vi "PID with MFC Challenge.vi"(8 "error in":errorcluster, 11 "classes in":T1) -> (0 "error out":errorcluster, 3 "classes out":T1)   [LabVIEW 2011]
uses:
  Controls/Class Objects.ctl
  Modules/File/Configuration/Configuration.lvclass
  Modules/Hardware/Power Supply/Power Supply.lvclass
  Modules/Hardware/Mass Flow Controller/Mass Flow Controller.lvclass
  Modules/Hardware/PID/PID.lvclass
  Modules/Hardware/Valve Controller/Valve Controller.lvclass
  Modules/Hardware/Multimeter/Multimeter.lvclass
  Modules/Hardware/Vapour Generator/Vapour Generator.lvclass
  Modules/File/TDMS/TDMS.lvclass
  Controls/User Interface Action.ctl
  Functional Global Data/Device Params Global.ctl
  Functional Global Data/Run Data.ctl
  Controls/TDMS File Handling.ctl
  <vilib>/Platform/TimedLoop/XDataNode/timing_clust.ctl
  <vilib>/Platform/TimedLoop/XDataNode/nitl_modes.ctl
  <vilib>/Platform/TimedLoop/XDataNode/wakeup.ctl
  Modules/File/TDMS/File Level.ctl
  <vilib>/Platform/TimedLoop/XDataNode/XDataNode.xnode
  <vilib>/Platform/TimedLoop/XDataNode/XDNodeRunTimeDep.lvlib
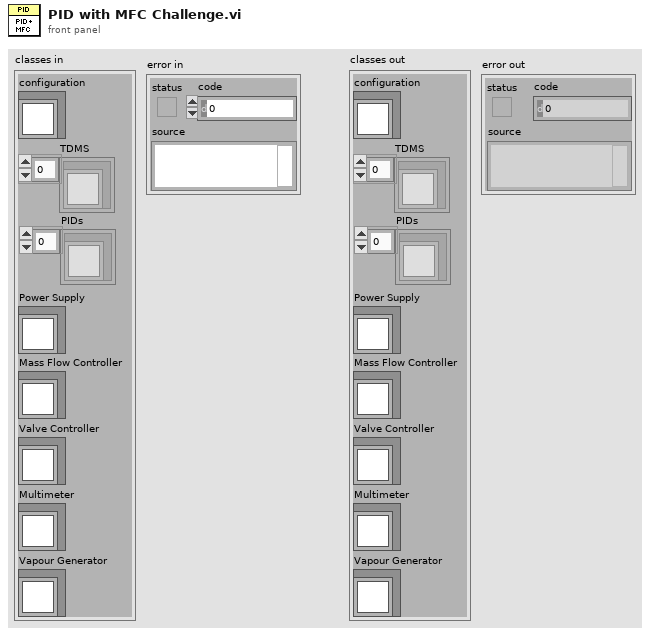
[diagram p1: front panel]
types:
  T1 = typedef "Class Objects.ctl" = cluster{"configuration":refnum<class "Configuration.lvclass">, "TDMS":refnum<class "TDMS.lvclass">[], "Power Supply":refnum<class "Power Supply.lvclass">, "Mass Flow Controller":refnum<class "Mass Flow Controller.lvclass">, "Valve Controller":refnum<class "Valve Controller.lvclass">, "Multimeter":refnum<class "Multimeter.lvclass">, "Vapour Generator":refnum<class "Vapour Generator.lvclass">, "PIDs":refnum<class "PID.lvclass">[]}
  T2 = typedef "User Interface Action.ctl" = enum16{"Initialize", "Data Acquisition Disable", "Data View Disable", "Sample Set", "Sample Set 2D Data", "Sample Set x0 & dx", "Sample Add", "Sample Set Cursor", "Sample Set Offset & Multiplier", "Sample Set Axis Labels", "Sample Parameters Disabled", "Sample Parameters Update", "Run Update", "Run Set Offset & Multiplier", "Run Set Axis Labels", "Run Set Cursor", "Run Set Disabled", "Run Parameters Update", "Run Parameters Disabled", "Run Number Set", "Run Number Set Range", "Run Number Set Disabled", "Sample Number Set", "Sample Number Set Range", "Notes Set Value", "Update Plot", "Set Plot Parameters", "Update Concentration Plot", "Time Set", "Clear DAQ Display", "Clear Analysis Display", "Status Bar Set", "Progress Bar Set", "Display Mode Set", "Experiment Type Set", "Analysis Plot Average Set", "Stop"}
  T3 = typedef "Device Params Global.ctl" = enum16{"Initialize", "Get Device Settings", "Get Device Connections", "Set Device Settings", "Set Device Connections", "Get All Device Properties"}
  T4 = typedef "Run Data.ctl" = enum16{"Initialize", "Add Sample Channel", "Set Run", "Get Number of Runs", "Set Run Params", "Get Spectrum", "Get Run Params", "Get Sample Params", "Get History", "Get Averaged History", "Get Run Param Names", "Set Run Param Names", "Get Sample Param Names", "Set Sample Param Names", "Get MFC Flow Rate Challenge Profile", "Get History Average"}
  T5 = typedef "TDMS File Handling.ctl" = enum16{"Add TDMS File", "Get Active TDMS File", "Set Active TDMS File", "Set Active TDMS File Index"}
  T6 = typedef "TDMS.lvclass/File Level.ctl" = enum16{"File", "Group", "Channel"}
  T7 = typedef "XDNodeRunTimeDep.lvlib/timing_clust.ctl" = cluster{"Expected End [f-1]":u64, "Actual End [f-1]":u64, "Finished Late? [f-1]":bool, "Expected End [i-1]":u64, "Actual End [i-1]":u64, "Finished Late? [i-1]":bool, "Expected Start [i]":u64, "Actual Start [i]":u64, "Expected Start [f]":u64, "Actual Start [f]":u64, "Source Name":string, "Structure Name":string, "Period":i64, "Deadline":i64, "Offset":i64, "Start":i64, "Priority":i32, "Timeout":i32, "Mode":T8, "Wakeup Reason":T9, "Error":errorcluster, "Source Type":string, "Secondary Source Type":string, "Global End Time":u64, "Global Start Time":u64, "Frame Duration":u64, "Iteration Duration":u64, "Assigned CPU":i32, "I/O Scan Engine Mode":u32}
  T8 = typedef "XDNodeRunTimeDep.lvlib/nitl_modes.ctl" = enum32{"No Change", "Process missed periods, maintain original phase", "Discard missed periods, maintain original phase", "Process missed periods, ignore original phase", "Discard missed periods, ignore original phase"}
  T9 = typedef "XDNodeRunTimeDep.lvlib/wakeup.ctl" = enum32{"Normal", "Aborted", "Asynchronous wakeup", "Timing source error", "Timed loop error", "Timeout"}
  T10 = typedef "Device Settings.ctl" = cluster{"PID":cluster{"B-M PID":T11, "INL PID":T12}, "Power Supply":cluster{"Source Value":dbl, "Source Value Units":T13, "Source Mode":T14, "Limits":T15, "Output":bool}, "Mass Flow Controller":cluster{"MFC Flow Rate":dbl, "MFC Valve Status":T18}, "Valve Controller":cluster{"Valve Assembly":T19}, "Multimeter":cluster{"Agilent 3458A":cluster{"Measurement Configuration":T21, "Measurement Integration":T22}}, "Vapour Generator":cluster{"Owlstone Permeation Tube":T23, "Owlstone GEN-SYS Setpoints":T25}}
  T11 = typedef "Baseline Mocon piD-Tech plus.lvclass/Settings.ctl" = cluster{"Detector Sampling Frequency":dbl}
  T12 = typedef "INL PID.lvclass/Settings.ctl" = cluster{"Sampling Frequency":dbl, "Integration Time":dbl, "Integration Periods":u8, "Grid Voltage":dbl}
  T13 = typedef "Power Supply.lvclass/Source Units.ctl" = enum16{"volts", "millivolts", "microvolts", "amps", "milliamps", "microamps", "nanoamps"}
  T14 = typedef "Power Supply.lvclass/Source Mode.ctl" = enum16{"Volts", "Current"}
  T15 = typedef "Power Supply.lvclass/Protection Limits.ctl" = cluster{"Voltage Limit":dbl, "Voltage Limit Units":T16, "Current Limit":dbl, "Current Limit Units":T17, "Voltage Trip/Cmpl":dbl, "Voltage Trip/Cmpl Units":T16, "Current Trip/Cmpl":dbl, "Current Trip/Cmpl Units":T17}
  T16 = typedef "Power Supply.lvclass/Voltage Units.ctl" = enum16{"volts", "millivolts", "microvolts"}
  T17 = typedef "Power Supply.lvclass/Current Units.ctl" = enum16{"amps", "milliamps", "microamps", "nanoamps"}
  T18 = typedef "Mass Flow Controller.lvclass/Valve Status.ctl" = enum16{"Open", "Closed"}
  T19 = typedef "Valve Controller.lvclass/Valve Assembly.ctl" = cluster{"Valve 1":T20, "Valve 2":T20, "Valve 3":T20, "Valve 4":T20, "Valve 5":T20}
  T20 = typedef "Valve Controller.lvclass/Status.ctl" = u16
  T21 = typedef "Agilent 3458A.lvclass/Measurement Configuration.ctl" = cluster{"Function":enum16{"DC Voltage", "AC Voltage", "AC + DC Voltage", "DC Current", "AC Current", "AC + DC Current", "2-Wire Resistance", "4-Wire Resistance", "Frequency", "Period", "Direct Sampling DC", "Direct Sampling AC", "Sub-Sampling DC", "Sub-Sampling AC"}, " Manual Resolution":enum16{"4.5", "5.5", "6.5", "7.5", "8.5"}, "Frequency Source":enum16{"AC + DC Current", "AC + DC Voltage", "AC Current", "AC Voltage"}, "Auto Range":enum16{"OFF", "ON", "ONCE"}}
  T22 = typedef "Agilent 3458A.lvclass/Measurement Integration.ctl" = cluster{"Power Line Cycles":dbl}
  T23 = typedef "Owlstone GEN-SYS.lvclass/Permeation Tube.ctl" = cluster{"Tube":T24, "Molecular Weight":dbl, "Calibration Temperature\n(Celcius)":i32, "Permeation Rate \n(ng/min)":i32}
  T24 = typedef "Owlstone GEN-SYS.lvclass/Permeation Tube Gas.ctl" = enum16{"Isobutylene 27 Nov 2012", "Ammonia 29 Sep 2012", "DMMP Tube A 3 July 2014", "DMMP Tube B 3 July 2014"}
  T25 = typedef "Owlstone GEN-SYS.lvclass/Gen-Sys Setpoints.ctl" = cluster{"OVG-4":cluster{"Oven Temperature":i32, "Sample Flow Rate":i32, "Split Flow Status":u16, "Split Flow Rate":i32}, "OHG-4":cluster{"Wet Air Flow":i32}}
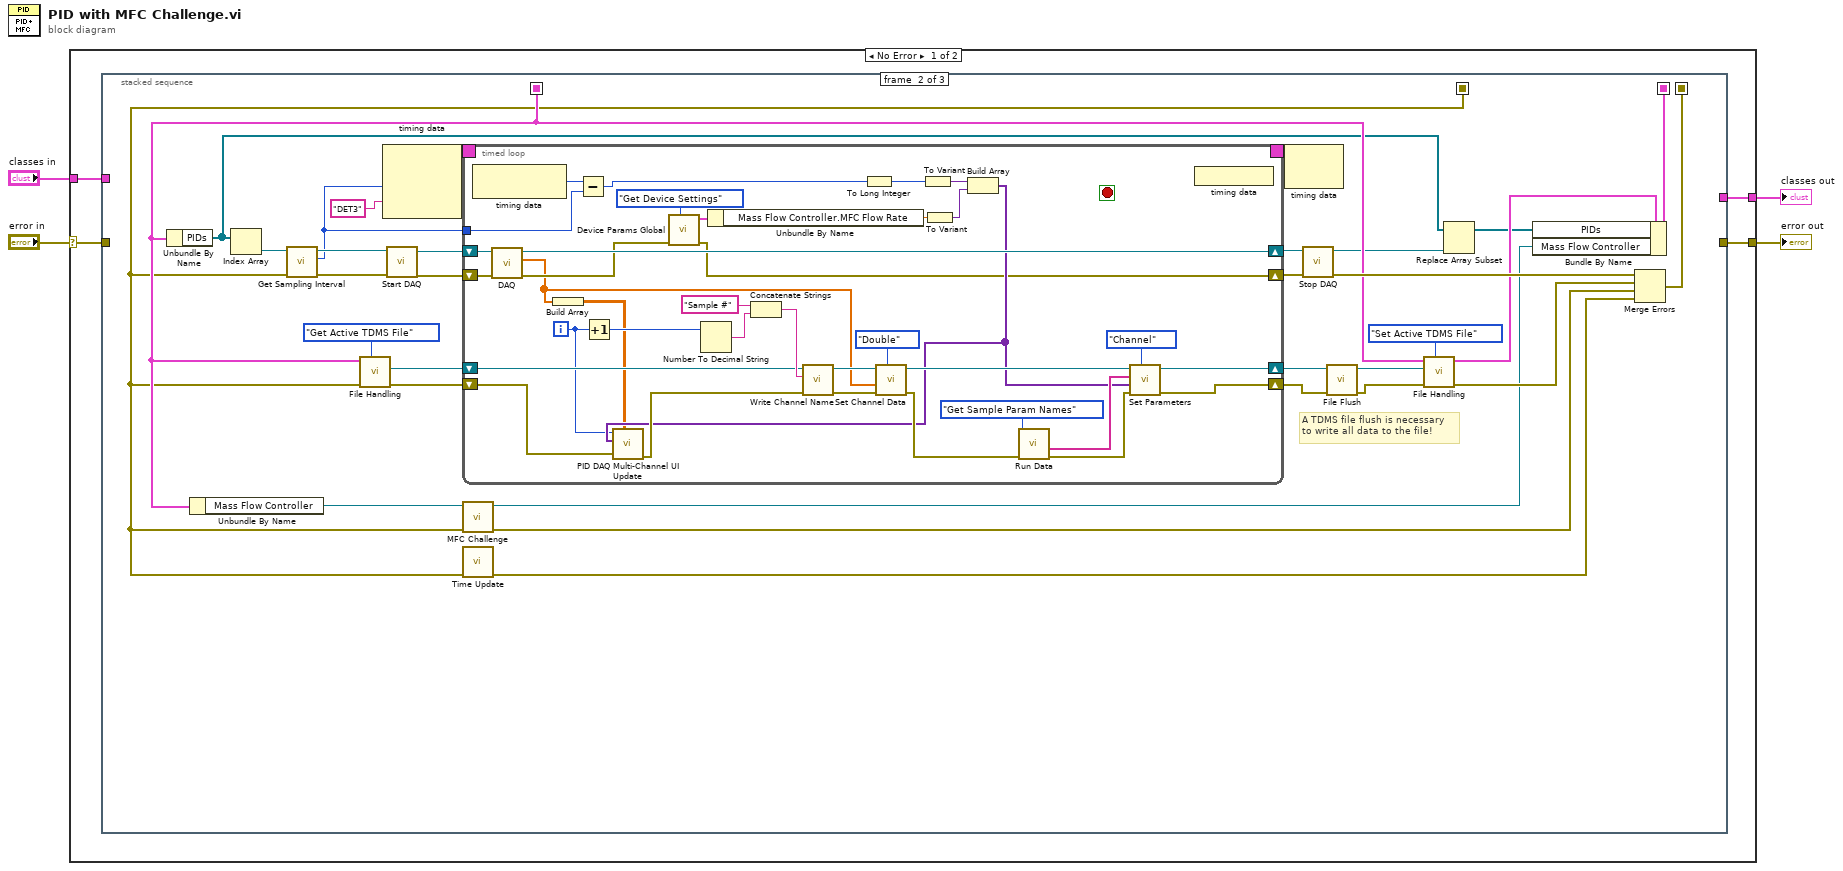
[diagram p0: block diagram]
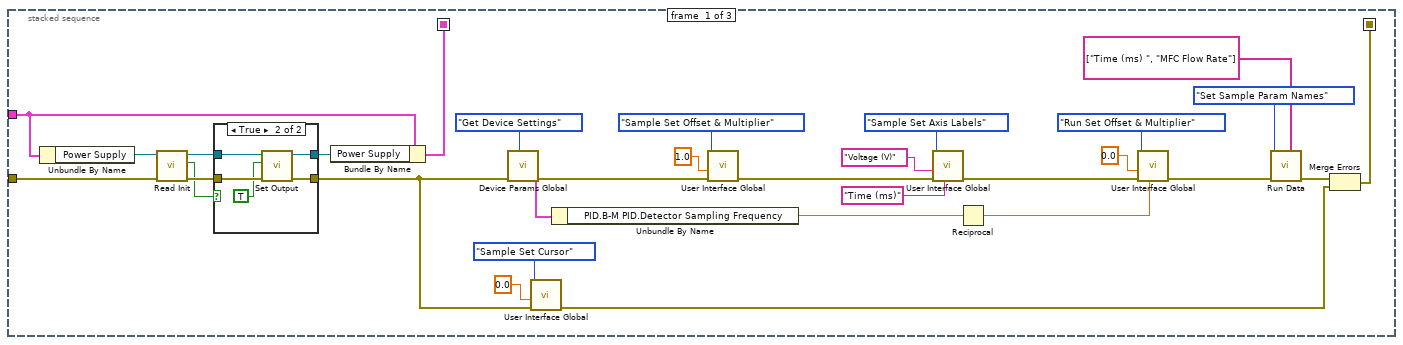
[diagram p2: hidden frame]
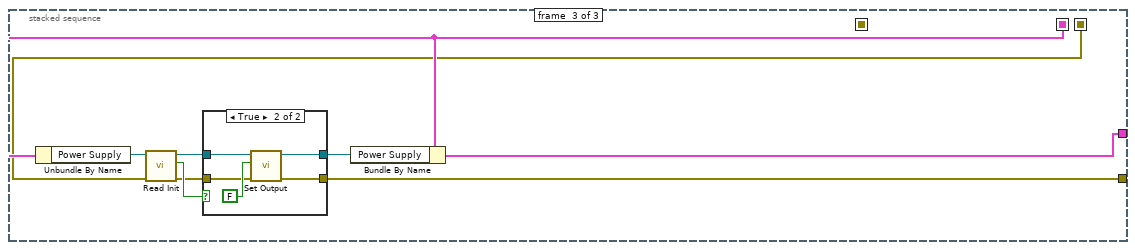
[diagram p4: hidden frame]
diagram:
  n1 = case shown="No Error" "error in" {
    selector: "error in" -> [w7 w140]
    tunnel: [w5 w140] -> w4
    tunnel: "classes in" -> [w8 w139]
    tunnel: [w6 w139] -> w1
    frame No Error {
      n2 = stacked-sequence {
        seq-local: [w32 _ _] -> [_ w60 _]
        seq-local: [w9 _ _] -> [_ w53 _]
        seq-local: [_ w59 _] -> [_ _ w126]
        seq-local: [_ w58 _] -> [_ _ w125]
        tunnel: w8 -> [w34 _ _]
        tunnel: w7 -> [w38 _ _]
        tunnel: [_ _ w127] -> w6
        tunnel: [_ _ w123] -> w5
        frame #0 {
          n3 = Unbundle By Name(w34) -> ("Power Supply"=w37:refnum<class "Power Supply.lvclass">)
          n4 = call-dynamic "Read Init.vi"("Power Supply in"=w37) -> ("Init"=w35:bool, "Power Supply out"=w36:refnum<class "Power Supply.lvclass">)  [unwired: 8 in, 1 out]
          n5 = case shown="True" w35 {
            tunnel: w38 -> [w39 w45]
            tunnel: w36 -> [w40 w44]
            tunnel: [w39 w41] -> w12
            tunnel: [w40 w42] -> w33
            frame False {
            }
            frame True {
              n6 = call-dynamic "Set Output.vi"("error in (no error)"=w45, "Enable"=TRUE, "Power Supply in"=w44) -> ("error out"=w41:errorcluster, "Power Supply out"=w42:refnum<class "Power Supply.lvclass">)  [unwired: 7 in]
            }
          }
          n7 = Bundle By Name(cluster=w34, "Power Supply"=w33) -> (w32:T1)
          n8 = call "Device Params Global.vi"("action"=Device_Params_Global."Get Device Settings", "error in"=w12) -> ("error out"=w17:errorcluster, "Device Settings OUT"=w18:T10)  [unwired: 7 in, 1 out]
          n9 = call "User Interface Global.vi"("error in"=w12, "data1"=0.0 ("1/x"), "action"=User_Interface_Action."Sample Set Cursor" ("Action")) -> ("error out"=w10:errorcluster)  [unwired: 8 in]
          n10 = Unbundle By Name(w18) -> ("PID.B-M PID.Detector Sampling Frequency"=w27:dbl)
          n11 = call "User Interface Global.vi"("error in"=w17, "data1"=1.0, "action"=User_Interface_Action."Sample Set Offset & Multiplier" ("Action")) -> ("error out"=w23:errorcluster)  [unwired: 8 in]
          n12 = call "User Interface Global.vi"("data2"="Time (ms)", "error in"=w23, "data1"="Voltage (V)", "action"=User_Interface_Action."Sample Set Axis Labels" ("Action")) -> ("error out"=w28:errorcluster)  [unwired: 7 in]
          n13 = Reciprocal(x=w27) -> (1/x=w16:dbl)
          n14 = call "User Interface Global.vi"("data2"=w16, "error in"=w28, "data1"=0.0 ("1/x"), "action"=User_Interface_Action."Run Set Offset & Multiplier" ("Action")) -> ("error out"=w15:errorcluster)  [unwired: 7 in]
          n15 = call "Run Data.vi"("Param Names IN"=string[] ["Time (ms) ", "MFC Flow Rate"] ("Sample Parm Names"), "error in"=w15, "action"=Run_Data."Set Sample Param Names") -> ("error out"=w11:errorcluster)  [unwired: 5 in, 3 out]
          n16 = Merge Errors(w11, w10) -> (w9:errorcluster)
        }
        frame #1 {
          # "A TDMS file flush is necessary\nto write all data to the file!"
          n17 = Unbundle By Name(w60) -> ("PIDs"=w46:refnum<class "PID.lvclass">[])
          n18 = Unbundle By Name(w60) -> ("Mass Flow Controller"=w57:refnum<class "Mass Flow Controller.lvclass">)
          n19 = Index Array(array=w46) -> (element=w49:refnum<class "PID.lvclass">)  [unwired: 1 in]
          n20 = call-dynamic "Get Sampling Interval.vi"("error in (no error)"=w53, "PID in"=w49) -> ("error out"=w51:errorcluster, "Sampling Interval"=w50:u32, "PID out"=w52:refnum<class "PID.lvclass">)  [unwired: 7 in]
          n21 = call "File Handling.vi"("TDMS File Handling"=TDMS_File_Handling."Get Active TDMS File", "error in"=w53, "Class objects"=w60) -> ("error out"=w68:errorcluster, "TDMS File"=w73:refnum<class "TDMS.lvclass">)  [unwired: 6 in, 1 out]
          n22 = node-c288(w50, "DET3" ("Name")) -> (w78:T7)  [unwired: 1 in]
          n23 = call-dynamic "Start DAQ.vi"("error in (no error)"=w51, "Detector in"=w52) -> ("error out"=w65:errorcluster, "Detector out"=w66:refnum<class "PID.lvclass">)  [unwired: 8 in]
          n24 = timed-loop {
            timing: w78 -> [_]
            timing-out: [_] -> w77
            shift-right: [w112] -> w64
            shift-left: w66 -> [w114]
            shift-right: [w96] -> w71
            shift-left: w68 -> [w100]
            shift-right: [w86] -> w72
            shift-left: w73 -> [w101]
            shift-right: [w87] -> w63
            shift-left: w65 -> [w113]
            tunnel: w50 -> [w83]
            i -> [w81]
            stop <- _ stop-if-true
            n25 = node-c288() -> (w84:i64)  [unwired: 1 in]
            n26 = call-dynamic "DAQ.vi"("error in"=w113, "Detector in"=w114) -> ("error out"=w90:errorcluster, "data"=w80:dbl[], "Detector out"=w112:refnum<class "PID.lvclass">)  [unwired: 7 in]
            n27 = Build Array(w80) -> (w79:dbl[][])
            n28 = Subtract(x=w84, y=w83) -> (x-y=w82:i64)
            n29 = Increment(x=w81) -> (x+1=w89:i32)
            n30 = call "Device Params Global.vi"("action"=Device_Params_Global."Get Device Settings", "error in"=w90) -> ("error out"=w87:errorcluster, "Device Settings OUT"=w91:T10)  [unwired: 7 in, 1 out]
            n31 = Number To Decimal String(number=w89) -> (decimal integer string=w102:string)  [unwired: 1 in]
            n32 = Unbundle By Name(w91) -> ("Mass Flow Controller.MFC Flow Rate"=w92:dbl)
            n33 = Concatenate Strings("Sample #" ("string"), w102) -> (w104:string)
            n34 = To Long Integer(number=w82) -> (32bit integer=w95:i32)
            n35 = To Variant(anything=w95) -> (Variant=w94:variant)
            n36 = To Variant(anything=w92) -> (Variant=w93:variant)
            n37 = Build Array(w94, w93) -> (w88:variant[])
            n38 = call "PID DAQ Multi-Channel UI Update.vi"("Sample Data"=w79, "error in"=w100, "Sample Parameter"=w88, "Sample Number"=w81) -> ("error out"=w99:errorcluster)  [unwired: 7 in]
            n39 = call-dynamic "Write Channel Name.vi"("error in (no error)"=w99, "Channel Name"=w104, "TDMS in"=w101) -> ("error out"=w109:errorcluster, "TDMS out"=w106:refnum<class "TDMS.lvclass">)  [unwired: 7 in]
            n40 = call-dynamic "Set Channel Data.vi"("data type"=enum16{"I16", "Double"}."Double" ("Data Type"), "error in"=w109, "double channel data"=w80, "TDMS in"=w106) -> ("error out"=w98:errorcluster, "TDMS out"=w107:refnum<class "TDMS.lvclass">)  [unwired: 6 in]
            n41 = call "Run Data.vi"("error in"=w98, "action"=Run_Data."Get Sample Param Names" ("Action")) -> ("error out"=w97:errorcluster, "Param Names OUT"=w111:string[])  [unwired: 6 in, 2 out]
            n42 = call-dynamic "Set Parameters.vi"("File Level"=File_Level."Channel", "error in (no error)"=w97, "property values"=w88, "property names"=w111, "TDMS.lvclass in"=w107) -> ("error out"=w96:errorcluster, "TDMS.lvclass out"=w86:refnum<class "TDMS.lvclass">)  [unwired: 5 in]
            n43 = node-c288() -> ()  [unwired: 1 out]
          }
          n44 = call "MFC Challenge.vi"("error in"=w53, "Mass Flow Controller in"=w57) -> ("error out"=w55:errorcluster, "Mass Flow Controller out"=w56:refnum<class "Mass Flow Controller.lvclass">)  [unwired: 8 in]
          n45 = call "Time Update.vi"("error in"=w53) -> ("error out"=w54:errorcluster)  [unwired: 10 in]
          n46 = node-c288(w77) -> ()  [unwired: 1 out]
          n47 = call-dynamic "Stop DAQ.vi"("error in (no error)"=w63, "Detector in"=w64) -> ("error out"=w62:errorcluster, "Detector out"=w48:refnum<class "PID.lvclass">)  [unwired: 8 in]
          n48 = call-dynamic "File Flush.vi"("error in"=w71, "TDMS in"=w72) -> ("error out"=w70:errorcluster, "TDMS out"=w69:refnum<class "TDMS.lvclass">)  [unwired: 8 in]
          n49 = call "File Handling.vi"("TDMS File Handling"=TDMS_File_Handling."Set Active TDMS File", "error in"=w70, "TDMS File"=w69, "Class objects"=w60) -> ("error out"=w67:errorcluster, "Class objects"=w61:T1)  [unwired: 5 in, 1 out]
          n50 = Replace Array Subset(array=w46, new element=w48) -> (w47:refnum<class "PID.lvclass">[])  [unwired: 1 in]
          n51 = Bundle By Name(cluster=w61, "PIDs"=w47, "Mass Flow Controller"=w56) -> (w59:T1)
          n52 = Merge Errors(w62, w67, w55, w54) -> (w58:errorcluster)
        }
        frame #2 {
          n53 = Unbundle By Name(w126) -> ("Power Supply"=w131:refnum<class "Power Supply.lvclass">)
          n54 = call-dynamic "Read Init.vi"("error in (no error)"=w125, "Power Supply in"=w131) -> ("error out"=w124:errorcluster, "Init"=w129:bool, "Power Supply out"=w130:refnum<class "Power Supply.lvclass">)  [unwired: 7 in]
          n55 = case shown="True" w129 {
            tunnel: w124 -> [w132 w134]
            tunnel: w130 -> [w133 w138]
            tunnel: [w132 w136] -> w123
            tunnel: [w133 w135] -> w128
            frame False {
            }
            frame True {
              n56 = call-dynamic "Set Output.vi"("error in (no error)"=w134, "Enable"=FALSE, "Power Supply in"=w138) -> ("error out"=w136:errorcluster, "Power Supply out"=w135:refnum<class "Power Supply.lvclass">)  [unwired: 7 in]
            }
          }
          n57 = Bundle By Name(cluster=w126, "Power Supply"=w128) -> (w127:T1)
        }
      }
    }
    frame Error {
    }
  }
  "error out" <- w4
  "classes out" <- w1
